vi "_TEST Users.vi"(4 "error in (no error)":errorcluster) -> (0 "error out":errorcluster)   [LabVIEW 2011]
uses:
  User Record.ctl
panel:
  out "User":T1
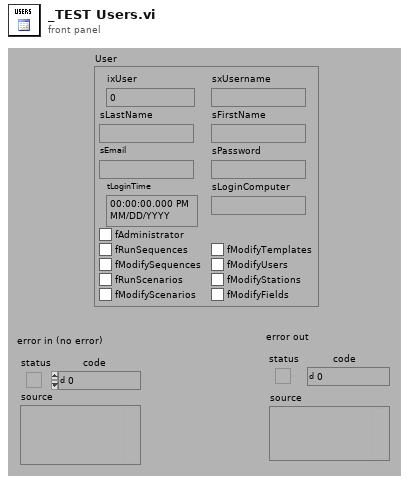
[diagram p1: front panel]
types:
  T1 = typedef "User Record.ctl" = cluster{"ixUser":i32, "sxUsername":string, "sLastName":string, "sFirstName":string, "sEmail":string, "sPassword":string, "tLoginTime":timestamp, "sLoginComputer":string, "fAdministrator":bool, "fRunSequences":bool, "fModifySequences":bool, "fRunScenarios":bool, "fModifyScenarios":bool, "fModifyTemplates":bool, "fModifyUsers":bool, "fModifyStations":bool, "fModifyFields":bool}
  T2 = typedef "Connection Refnum.ctl" = cluster{"Environment Handle":i32, "Connection Handle":i32}
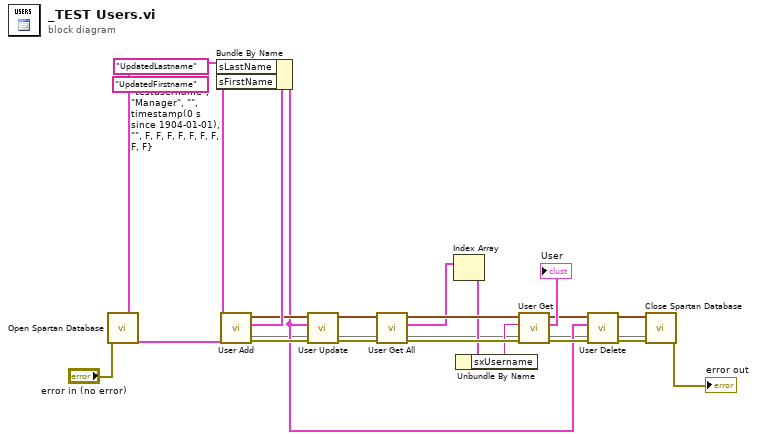
[diagram p0: block diagram]
diagram:
  n1 = call "Open Spartan Database.vi"("error in (no error)"="error in (no error)") -> ("error out"=w24:errorcluster, "Connection Refnum"=w23:T2, 4:w3)  [unwired: 1 in, 7 out]
  n2 = call "User Add.vi"("error in (no error)"=w24, "User Record"=T1 {"ixUser"=0, "sxUsername"="Lastname", "sLastName"="Firstname", "sFirstName"="testusername", "sEmail"="Manager", "sPassword"="", "tLoginTime"=timestamp(0 s since 1904-01-01), "sLoginComputer"="", "fAdministrator"=FALSE, "fRunSequences"=FALSE, "fModifySequences"=FALSE, "fRunScenarios"=FALSE, "fModifyScenarios"=FALSE, "fModifyTemplates"=FALSE, "fModifyUsers"=FALSE, "fModifyStations"=FALSE, "fModifyFields"=FALSE} ("Users Information"), "Connection Refnum"=w23) -> ("error out"=w21:errorcluster, "New User Record"=w20:T1, "Connection Refnum"=w19:T2)  [unwired: 6 in]
  n3 = Bundle By Name(cluster=w20, "sLastName"="UpdatedLastname" ("Last Name"), "sFirstName"="UpdatedFirstname" ("Last Name")) -> (w6:T1)
  n4 = call "User Update.vi"("error in (no error)"=w21, "User Record"=w6, "Connection Refnum"=w19) -> ("error out"=w15:errorcluster, "dup Connection Refnum"=w16:T2)  [unwired: 7 in]
  n5 = call "User Get All.vi"("error in (no error)"=w15, "Connection Refnum"=w16) -> ("error out"=w13:errorcluster, "User Records"=w12:T1[], "Connection Refnum"=w14:T2)  [unwired: 6 in, 1 out]
  n6 = Index Array(array=w12) -> (element=w11:T1)  [unwired: 1 in]
  n7 = Unbundle By Name(w11) -> ("sxUsername"=w10:string)
  n8 = call "User Get.vi"("error in (no error)"=w13, "sxUsername (\"\")"=w10, "Connection Refnum"=w14) -> ("error out"=w7:errorcluster, "User"=→"User":T1, "Connection Refnum"=w8:T2)  [unwired: 5 in, 1 out]
  n9 = call "User Delete.vi"("error in (no error)"=w7, "User Record"=w6, "Connection Refnum"=w8) -> ("error out"=w4:errorcluster, "Connection Refnum"=w5:T2)  [unwired: 7 in]
  n10 = call "Close Spartan Database.vi"("Force Close? (f)"=w3, "error in (no error)"=w4, "Connection Refnum"=w5) -> ("error out"=→"error out":errorcluster)  [unwired: 1 in, 7 out]
